vi "Find Top Level Reference.vi"(8 "error in (no error)":errorcluster, 11 "String":string) -> (0 "error out":errorcluster, 3 "Ctl Refnum":refnum<vi>)   [LabVIEW 2020]
doc: "This software is licensed for use under the “MIT License\"\nCopyright (c) 2019 Scott Hannahs, sth@alum.mit.edu\n\nPermission is hereby granted, free of charge, to any person obtaining a copy of this software and associated documentation files (the \"Software\"), to deal in the Software without restriction, including without limitation the rights to use, copy, modify, merge, publish, distribute, sublicense, and/or sell copies of the Software, and to permit persons to whom the Software is furnished to do so, subject to the following conditions: The above copyright notice and this permission notice shall be included in all copies or substantial portions of the Software.\n\nTHE SOFTWARE IS PROVIDED \"AS IS\", WITHOUT WARRANTY OF ANY KIND, EXPRESS OR IMPLIED, INCLUDING BUT NOT LIMITED TO THE WARRANTIES OF MERCHANTABILITY, FITNESS FOR A PARTICULAR PURPOSE AND NONINFRINGEMENT. IN NO EVENT SHALL THE AUTHORS OR COPYRIGHT HOLDERS BE LIABLE FOR ANY CLAIM, DAMAGES OR OTHER LIABILITY, WHETHER IN AN ACTION OF CONTRACT, TORT OR OTHERWISE, ARISING FROM, OUT OF OR IN CONNECTION WITH THE SOFTWARE OR THE USE OR OTHER DEALINGS IN THE SOFTWARE."
uses:
  <vilib>/Utility/error.llb/Error Cluster From Error Code.vi
  <vilib>/ErrorRing/Error Ring.xnode
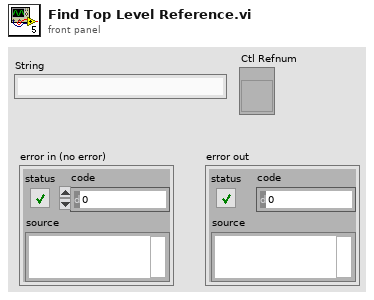
[diagram p1: front panel]
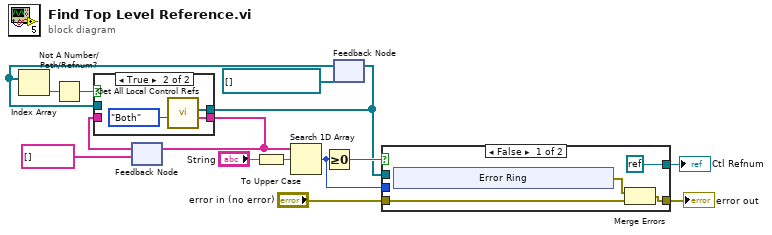
[diagram p0: block diagram]
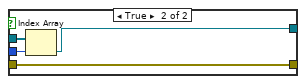
[diagram p3: hidden frame]
diagram:
  n1 = feedback #1(string[] [] ("Control Labels")) -> (w10:string[])
  n2 = To Upper Case(1:"String") -> (0:w4:string)
  n3 = feedback #2(refnum<vi>[] [] ("All Controls")) -> (w2:refnum<vi>[])
  n4 = Index Array(array=w2) -> (element=w3:refnum<vi>)  [unwired: 1 in]
  n5 = Not A Number/Path/Refnum?(number/path/refnum=w3) -> (NaN/Path/Refnum?=w1:bool)
  n6 = case shown="True" w1 {
    tunnel: [w17 w19] -> w9
    tunnel: w2 -> [w17 _]
    tunnel: [w16 w18] -> w8
    tunnel: w10 -> [w16 _]
    frame False {
    }
    frame True {
      n7 = call "Get All Local Control Refs.vi"("Type"=enum16{"Both", "Controls", "Indicators"}."Both") -> ("All Controls"=w19:refnum<vi>[], "Control Labels"=w18:string[])  [unwired: 4 in, 2 out]
    }
  }
  n8 = feedback-in #1(w8) -> ()
  n9 = Search 1D Array(1D array=w8, element=w4) -> (index of element=w12:i32)  [unwired: 1 in]
  n10 = Greater Or Equal To 0?(x=w12) -> (x >= 0?=w14:bool)
  n11 = feedback-in #2(w9) -> ()
  n12 = case shown="False" w14 {
    tunnel: [w24 w30] -> w11
    tunnel: "error in (no error)" -> [w23 w30]
    tunnel: w12 -> [_ w33]
    tunnel: w9 -> [_ w32]
    tunnel: [refnum<k0> refnum w31] -> w7
    frame False {
      n13 = xnode "Error Ring"() -> ("error out"=w22:errorcluster)
      n14 = Merge Errors(w22, w23) -> (w24:errorcluster)
    }
    frame True {
      n15 = Index Array(array=w32, index=w33) -> (element=w31:refnum<vi>)
    }
  }
  "error out" <- w11
  "Ctl Refnum" <- w7
